vi "UpdateFeatureStudio.vi"(0 "Device In":T1, 11 "error in":errorcluster, 12 "FeatureScript":string) -> (4 "Device Out":T1, 6 "Comm":T2, 15 "error out":errorcluster)   [LabVIEW 2019]
uses:
  <userlib>/IoT Devices/_subVIs/HTTPComm.ctl
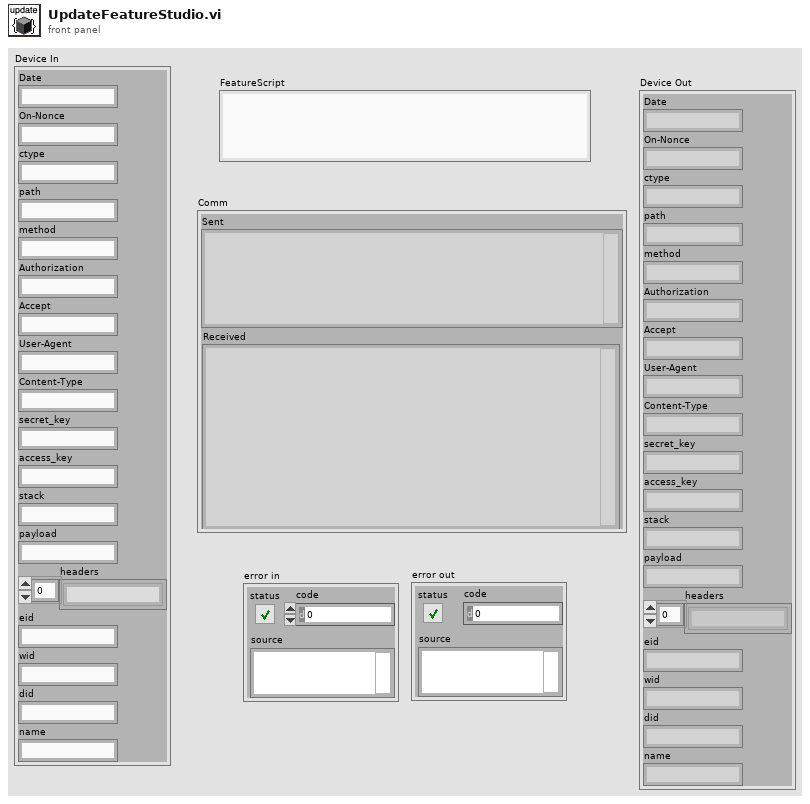
[diagram p1: front panel]
types:
  T1 = cluster{"Date":string, "On-Nonce":string, "ctype":string, "path":string, "method":string, "Authorization":string, "Accept":string, "User-Agent":string, "Content-Type":string, "secret_key":string, "access_key":string, "stack":string, "payload":string, "headers":string[], "eid":string, "wid":string, "did":string, "name":string}
  T2 = typedef "HTTPComm.ctl" = cluster{"url":string, "sent headers":string, "sent body":string, "headers":string, "body":string, "Sent":string, "Received":string}
  T3 = cluster{"contents":string, "serializationVersion":string, "sourceMicroversion":string, "rejectMicroversionSkew":bool}
  T4 = cluster{"contents":string, "serializationVersion":string, "sourceMicroversion":string, "rejectMicroversionSkew":bool, "microversionSkew":bool, "libraryVersion":i32}
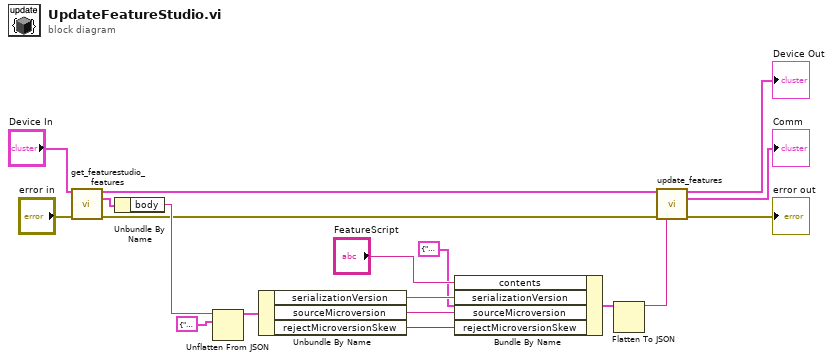
[diagram p0: block diagram]
diagram:
  n1 = call <userlib>:"get_featurestudio_features.vi"("Device In"="Device In", "error in"="error in") -> ("Device Out"=w3:T1, "Comm"=w4:T2, "error out"=w2:errorcluster)  [unwired: 11 in]
  n2 = Unbundle By Name(w4) -> ("body"=w10:string)
  n3 = Unflatten From JSON(JSON string=w10, type and defaults=T4 {"contents"="", "serializationVersion"="", "sourceMicroversion"="", "rejectMicroversionSkew"=TRUE, "microversionSkew"=TRUE, "libraryVersion"=0}) -> (value=w14:T4)  [unwired: 5 in, 1 out]
  n4 = Unbundle By Name(w14) -> ("serializationVersion"=w15:string, "sourceMicroversion"=w16:string, "rejectMicroversionSkew"=w17:bool)
  n5 = Bundle By Name(cluster=T3 {"contents"="", "serializationVersion"="", "sourceMicroversion"="", "rejectMicroversionSkew"=TRUE}, "contents"="FeatureScript", "serializationVersion"=w15, "sourceMicroversion"=w16, "rejectMicroversionSkew"=w17) -> (w12:T3)
  n6 = Flatten To JSON(anything=w12) -> (JSON string=w8:string)  [unwired: 2 in, 1 out]
  n7 = call <userlib>:"update_features.vi"("Device In"=w3, "error in"=w2, "Features"=w8) -> ("Device Out"=→"Device Out":T1, "Comm"=→"Comm":T2, "error out"=→"error out":errorcluster)  [unwired: 10 in]
